vi "analysis.vi"() -> ()   [LabVIEW 2019]
uses:
  <vilib>/vision/NI_Vision_Development_Module.lvlib
panel:
  out "XY Graph 5":cluster{dbl[], dbl[]}(graph)
  out "size(s)":i32
  out "XY Graph 3":cluster{dbl[], dbl[]}(graph)
  out "XY Graph 2":cluster{"Y":dbl[], "Y":dbl[]}[](graph)
  out "Array 2":path[](array[path])
  out "XY Graph":cluster{"Y":dbl[], "Y":dbl[]}[](graph)
  in  "directory path":path
  out "Array":path[][](array[path])
  in  "Range":cluster{"Lower value":sgl, "Upper value":sgl}={"Lower value"=128.0, "Upper value"=255.0} {"Upper value" format="%.2f"; "Lower value" format="%.2f"}
  out "Image":T1(plugin-control)
  in  "File Path":path
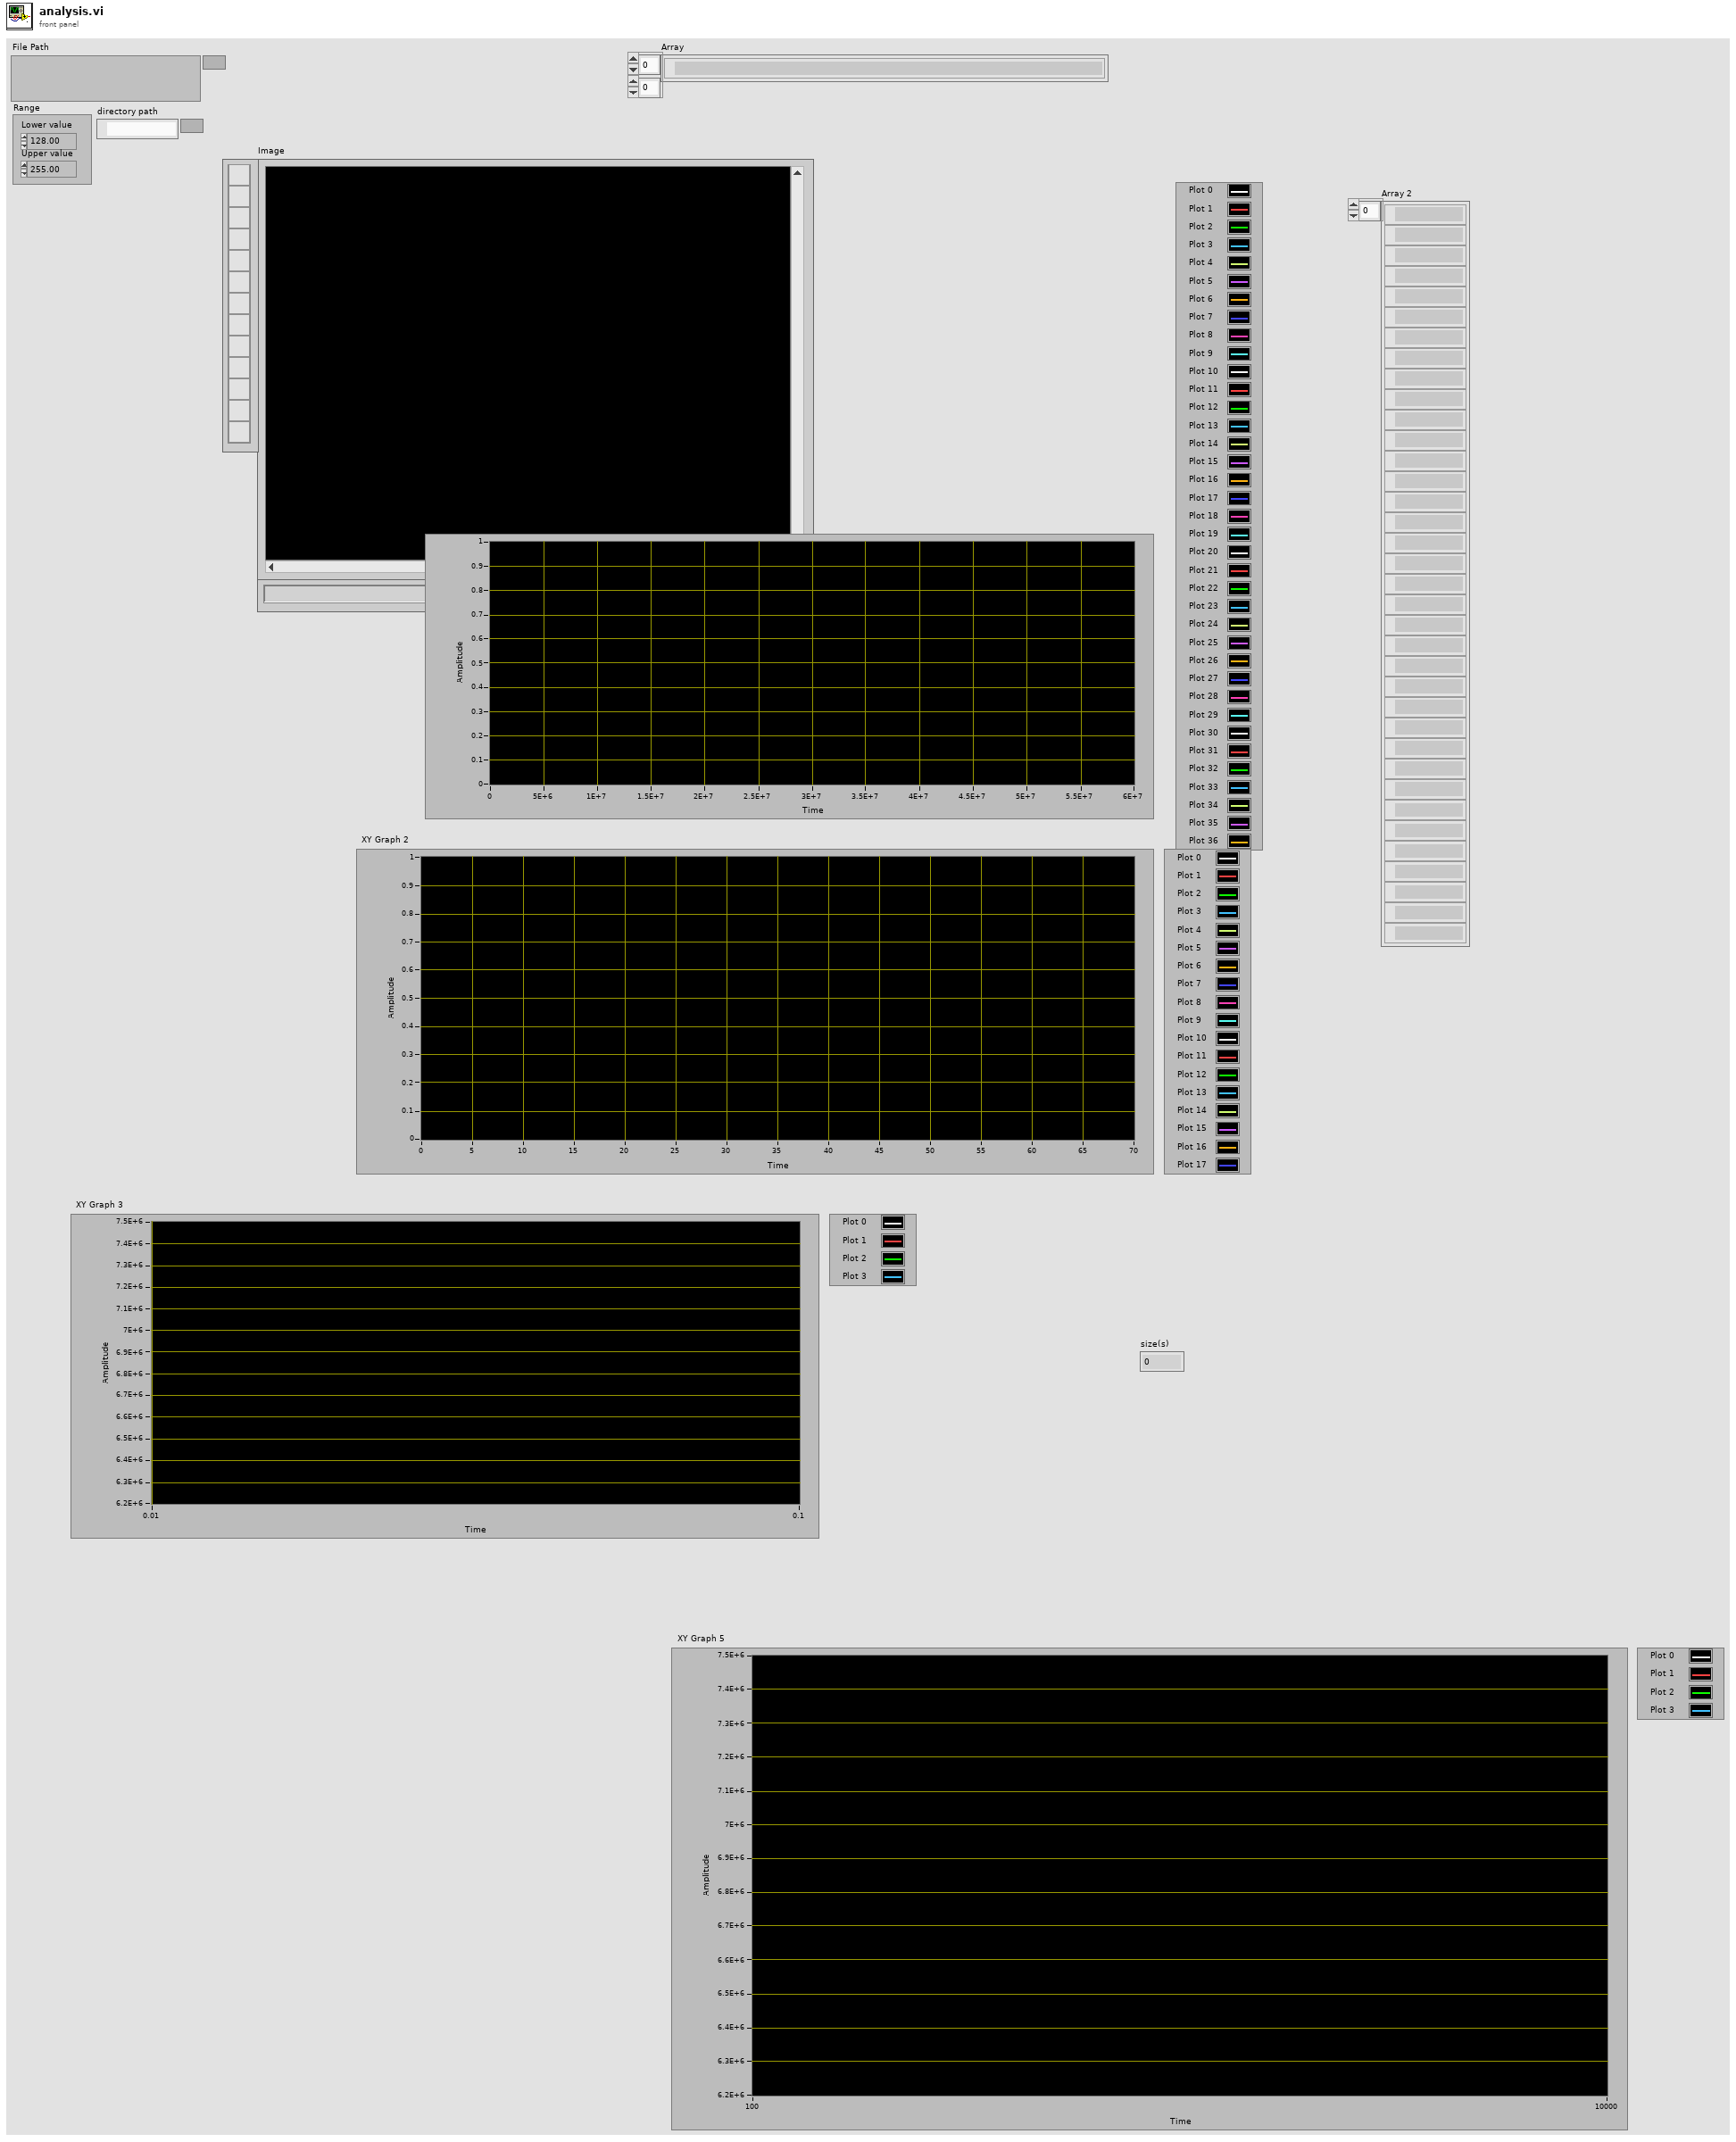
[diagram p1: front panel]
types:
  T1 = typedef "IMAQ Image.ctl" = refnum<image>
  T2 = typedef "LVDateTimeRec.ctl" = cluster{"fractional second":dbl, "second":i32, "minute":i32, "hour":i32, "day of month":i32, "month":i32, "year":i32, "day of week":i32, "day of year":i32, "DST":i32}
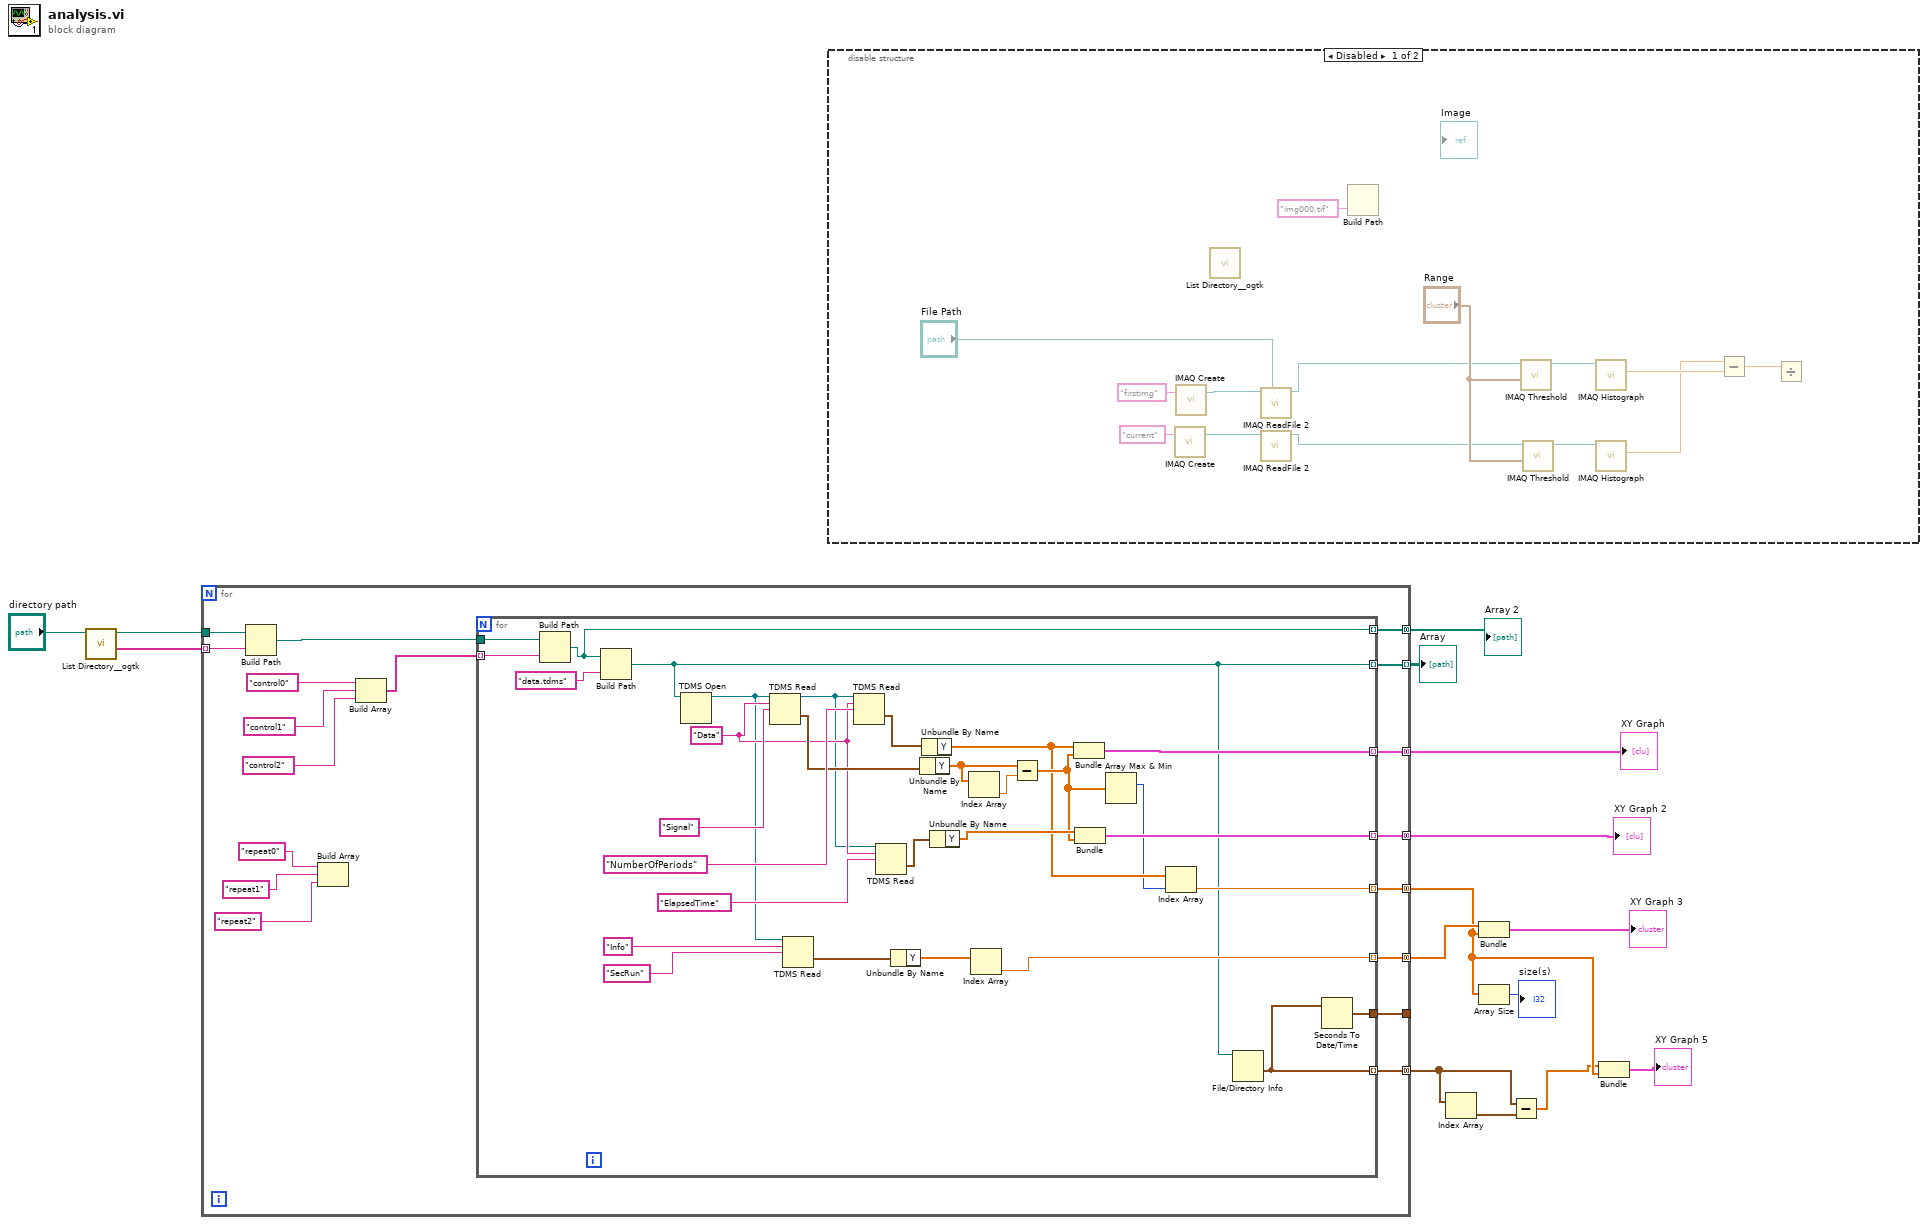
[diagram p0: block diagram]
diagram:
  n1 = call <userlib>:"List Directory__ogtk.vi"("directory path"="directory path") -> ("directory names"=w14:string[], "dup directory path"=w15:path)  [unwired: 3 in, 2 out]
  n2 = for {
    tunnel: w15 -> [w33]
    tunnel: w14 -> [w32] mode=indexing
    tunnel: [w31] -> w10 mode=concatenating
    tunnel: [w30] -> w13 mode=indexing
    tunnel: [w29] -> w11 mode=concatenating
    tunnel: [w20] -> w9 mode=concatenating
    tunnel: [w19] -> w4 mode=concatenating
    tunnel: [w18] -> w8 mode=concatenating
    tunnel: [w17] -> w2 mode=concatenating
    tunnel: [w16] -> _
    n3 = Build Path(base path=w33, name or relative path=w32) -> (appended path=w28:path)
    n4 = Build Array("repeat0" ("name or relative path"), "repeat1" ("name or relative path"), "repeat2" ("name or relative path")) -> ()  [unwired: 1 out]
    n5 = Build Array("control0" ("name or relative path"), "control1" ("name or relative path"), "control2" ("name or relative path")) -> (w24:string[])
    n6 = for {
      tunnel: w28 -> [w63]
      tunnel: w24 -> [w62] mode=indexing
      tunnel: [w60] -> w31 mode=indexing
      tunnel: [w36] -> w30 mode=indexing
      tunnel: [w55] -> w29 mode=indexing
      tunnel: [w50] -> w20 mode=indexing
      tunnel: [w43] -> w19 mode=indexing
      tunnel: [w37] -> w18 mode=indexing
      tunnel: [w34] -> w17 mode=indexing
      tunnel: [w35] -> w16
      w54 = "Data" ("group name in")
      n7 = Build Path(base path=w63, name or relative path=w62) -> (appended path=w60:path)
      n8 = Build Path(base path=w60, name or relative path="data.tdms" ("Image Name")) -> (appended path=w36:path)
      n9 = TDMS Open(11:w36) -> (3:w42:refnum<k34>)  [unwired: 6 in, 1 out]
      n10 = TDMS Read(0:w42, 5:w54, 7:"Signal" ("group name in")) -> (4:w49:refnum<k34>, 10:w56:waveform(dbl))  [unwired: 5 in, 4 out]
      n11 = TDMS Read(0:w42, 5:"Info" ("group name in"), 7:"SecRun" ("group name in")) -> (10:w39:waveform(dbl))  [unwired: 5 in, 5 out]
      n12 = TDMS Read(0:w49, 5:w54, 7:"NumberOfPeriods" ("group name in")) -> (10:w57:waveform(dbl))  [unwired: 5 in, 5 out]
      n13 = TDMS Read(0:w49, 5:w54, 7:"ElapsedTime" ("group name in")) -> (10:w52:waveform(dbl))  [unwired: 5 in, 5 out]
      n14 = Unbundle By Name(w39) -> ("Y"=w38:dbl[])
      n15 = Unbundle By Name(w56) -> ("Y"=w47:dbl[])
      n16 = Unbundle By Name(w57) -> ("Y"=w45:dbl[])
      n17 = Unbundle By Name(w52) -> ("Y"=w51:dbl[])
      n18 = Index Array(array=w47) -> (element=w48:dbl)  [unwired: 1 in]
      n19 = Index Array(array=w38) -> (element=w37:dbl)  [unwired: 1 in]
      n20 = Subtract(x=w47, y=w48) -> (x-y=w46:dbl[])
      n21 = Bundle("Y"=w45, w46) -> (w55:cluster{"Y":dbl[], dbl[]})  [unwired: 1 in]
      n22 = Bundle("Y"=w51, w46) -> (w50:cluster{"Y":dbl[], dbl[]})  [unwired: 1 in]
      n23 = Array Max & Min(array=w46) -> (max index (indices)=w44:i32)  [unwired: 3 out]
      n24 = Index Array(array=w45, index=w44) -> (element=w43:dbl)
      n25 = File/Directory Info(path=w36) -> (last mod=w34:timestamp)  [unwired: 1 in, 6 out]
      n26 = Seconds To Date/Time(time stamp (now)=w34) -> (date time rec=w35:T2)  [unwired: 1 in]
    }
  }
  "Array" <- w13
  "XY Graph" <- w11
  "Array 2" <- w10
  "XY Graph 2" <- w9
  n27 = disable-structure shown="Disabled" {
    frame Disabled {
      n28 = call "IMAQ Create"("Image Name"="current") -> ("New Image"=w67:T1)  [unwired: 4 in, 1 out]
      n29 = call "IMAQ Create"("Image Name"="firstimg") -> ("New Image"=w77:T1)  [unwired: 4 in, 1 out]
      n30 = call <userlib>:"List Directory__ogtk.vi"() -> ()  [unwired: 4 in, 4 out]
      n31 = call "IMAQ ReadFile 2"("File Path"="File Path", "Image"=w77) -> ("Image Out"=w66:T1)  [unwired: 5 in, 4 out]
      n32 = call "IMAQ ReadFile 2"("Image"=w67) -> ("Image Out"=w65:T1)  [unwired: 6 in, 4 out]
      n33 = Build Path(name or relative path="img000.tif") -> ()  [unwired: 1 in, 1 out]
      n34 = call "IMAQ Threshold"("Range"="Range", "Image Src"=w66) -> ("Image Dst Out"=w73:T1)  [unwired: 8 in, 1 out]
      n35 = call "IMAQ Threshold"("Range"="Range", "Image Src"=w65) -> ("Image Dst Out"=w69:T1)  [unwired: 8 in, 1 out]
      n36 = call "IMAQ Histograph"("Image"=w73) -> ("Mean Value"=w71:sgl)  [unwired: 7 in, 3 out]
      n37 = call "IMAQ Histograph"("Image"=w69) -> ("Mean Value"=w64:sgl)  [unwired: 7 in, 3 out]
      n38 = Subtract(x=w64, y=w71) -> (x-y=w72:sgl)
      n39 = Divide(x=w72) -> ()  [unwired: 1 in, 1 out]
    }
    frame Enabled {
    }
  }
  n40 = Index Array(array=w2) -> (element=w3:timestamp)  [unwired: 1 in]
  n41 = Bundle(w8, w4) -> (→"XY Graph 3":cluster{dbl[], dbl[]})  [unwired: 1 in]
  n42 = Array Size(array=w4) -> (size(s)=→"size(s)":i32)
  n43 = Subtract(x=w2, y=w3) -> (x-y=w1:dbl[])
  n44 = Bundle(w1, w4) -> (→"XY Graph 5":cluster{dbl[], dbl[]})  [unwired: 1 in]
